vi "sub_play_image_stream.vi"() -> ()   [LabVIEW 2014]
uses:
  <vilib>/vision/Image Controls.llb/IMAQ Image.ctl
panel:
  out "frame":T1
  in  "fps":u32
  in  "frame":string
  in  "frame num":u32
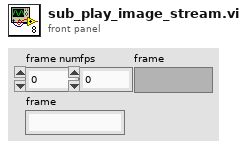
[diagram p1: front panel]
types:
  T1 = typedef "IMAQ Image.ctl" = refnum<image>
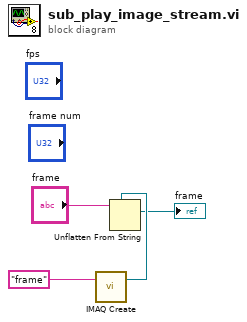
[diagram p0: block diagram]
diagram:
  n1 = call "IMAQ Create"("Image Name"="frame") -> ("New Image"=w2:T1)  [unwired: 4 in, 1 out]
  n2 = Unflatten From String(type=w2, binary string="frame") -> (value=→"frame":T1)  [unwired: 3 in, 2 out]
